vi "Set Polling Message.vi"(8 "error in (no error)":errorcluster, 10 "Polling Message":refnum<class "Message.lvclass">, 11 "OOQMH in":refnum<class "OOQMH.lvclass">) -> (0 "error out":errorcluster, 3 "OOQMH out":refnum<class "OOQMH.lvclass">)   [LabVIEW 2024, in "OOQMH.lvlib" / "OOQMH.lvclass"]
uses:
  OOQMH.lvclass
  OOQMH.lvclass/OOQMH.ctl
  Message/Message.lvclass
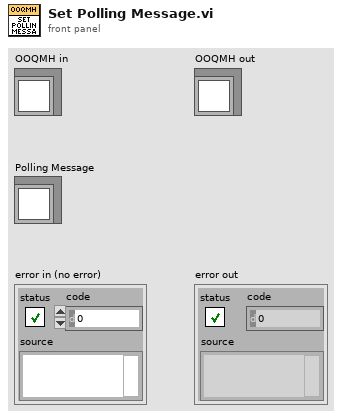
[diagram p1: front panel]
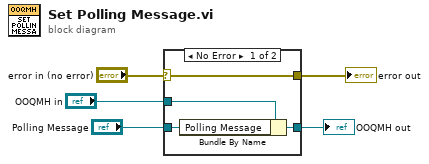
[diagram p0: block diagram]
diagram:
  n1 = case shown="No Error" "error in (no error)" {
    selector: "error in (no error)" -> [w9 w11]
    tunnel: [w9 w11] -> w4
    tunnel: [w7 w10] -> w2
    tunnel: "OOQMH in" -> [w8 w10]
    tunnel: "Polling Message" -> [w6 _]
    frame No Error {
      n2 = Bundle By Name(cluster=w8, "Polling Message"=w6) -> (w7:refnum<class "OOQMH.lvclass">)
    }
    frame Error {
    }
  }
  "error out" <- w4
  "OOQMH out" <- w2
